vi "CoboltLaser_ResponseCheck.vi"(0 "Response":string, 1 "ExpectedResponseType":T1 items=["Any", "Digits Only", "Non-Digits Only"], 2 "ExpectedResponseMinimumLength":i32 min=0 step=1, 3 "ErrorMessage":string, 4 "GenerateErrorIfFail":bool, 5 "ErrorIn":errorcluster) -> (15 "ResponseOK":bool, 16 "Retry":bool, 19 "ErrorOut":errorcluster)   [LabVIEW 2012, in "Cobolt.lvclass"]
doc: "Use this template to build a VI to use as a subVI."
uses:
  Template/Cobolt.lvclass
  CoboltLaser_Controls/ExpectedResponseType.ctl
  Instance           1 26Saved   PR59_ResponseCheck .vi
  <vilib>/regexp/Match Regular Expression.xnode
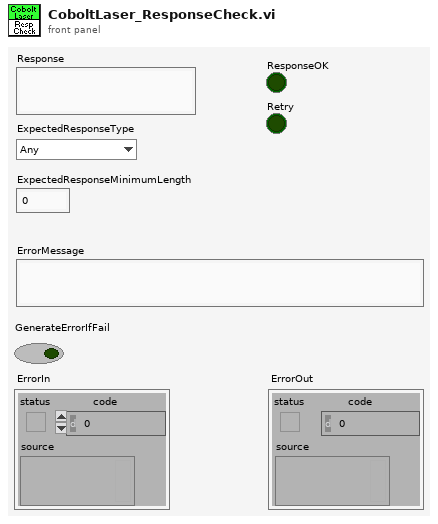
[diagram p1: front panel]
types:
  T1 = typedef "Cobolt.lvclass/ExpectedResponseType.ctl" = u16
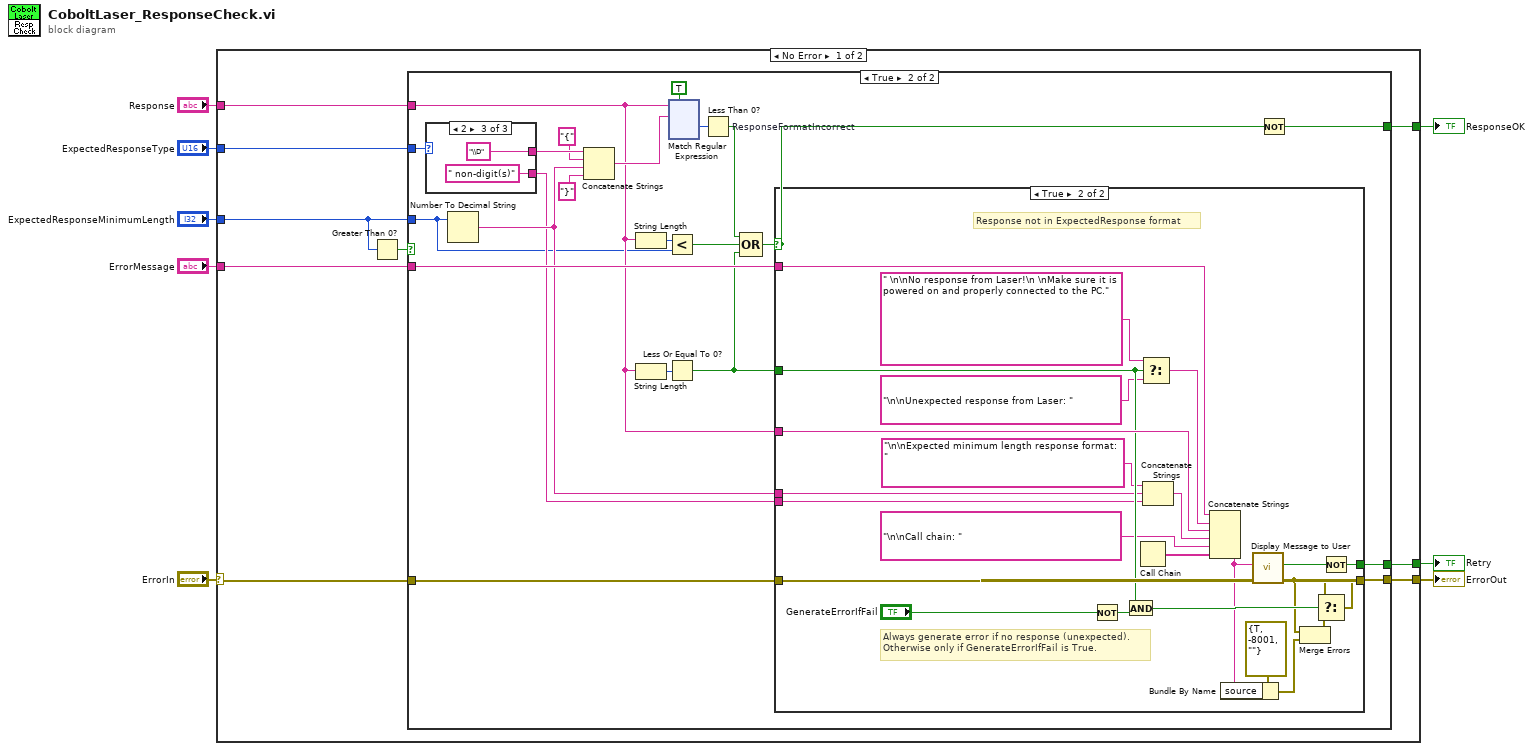
[diagram p0: block diagram]
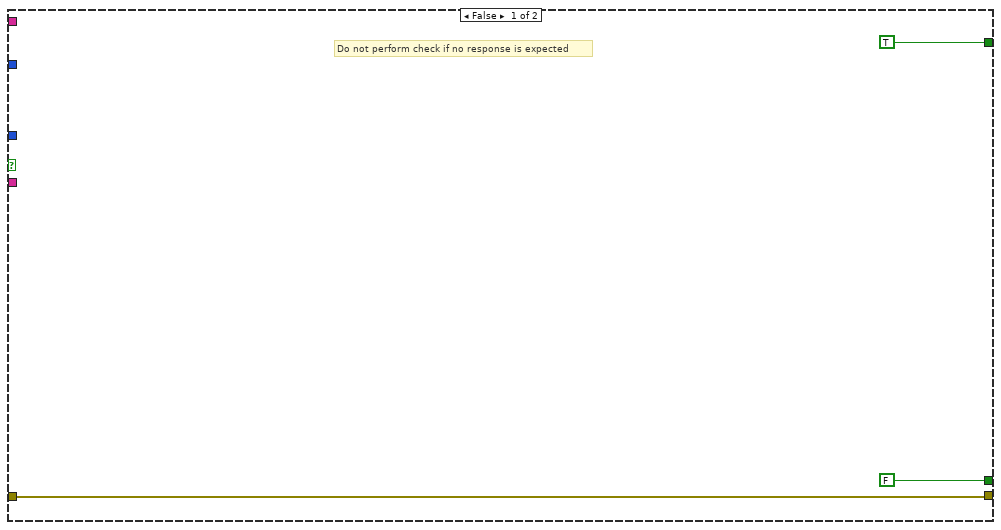
[diagram p2: hidden frame]
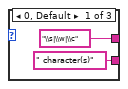
[diagram p3: hidden frame]
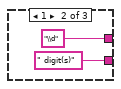
[diagram p4: hidden frame]
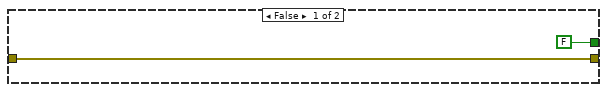
[diagram p5: hidden frame]
diagram:
  n1 = case shown="No Error" "ErrorIn" {
    selector: "ErrorIn" -> [w16 w186]
    tunnel: [w17 w186] -> w7
    tunnel: "ErrorMessage" -> [w14 _]
    tunnel: "ExpectedResponseMinimumLength" -> [w13 _]
    tunnel: "ExpectedResponseType" -> [w12 _]
    tunnel: "Response" -> [w11 _]
    tunnel: [w10 _] -> w2
    tunnel: [w9 _] -> w1
    frame No Error {
      n2 = Greater Than 0?(x=w13) -> (x > 0?=w15:bool)
      n3 = case shown="True" w15 {
        tunnel: [w18 w42] -> w17
        tunnel: w14 -> [_ w41]
        tunnel: w16 -> [w18 w40]
        tunnel: [FALSE w39] -> w9
        tunnel: w11 -> [_ w25]
        tunnel: w12 -> [_ w35]
        tunnel: w13 -> [_ w23]
        tunnel: [TRUE w29] -> w10
        frame False {
          # "Do not perform check if no response is expected"
        }
        frame True {
          n4 = case shown="2" w35 {
            tunnel: ["\\s|\\w|\\c" "\\d" "\\D"] -> w34
            tunnel: [" character(s)" " digit(s)" " non-digit(s)"] -> w27
            frame 0, Default {
            }
            frame 1 {
            }
            frame 2 {
            }
          }
          n5 = Number To Decimal String(number=w23) -> (decimal integer string=w28:string)  [unwired: 1 in]
          n6 = Concatenate Strings(w34, "{", w28, "}") -> (w31:string)
          n7 = String Length(string=w25) -> (length=w24:i32)
          n8 = String Length(string=w25) -> (length=w38:i32)
          n9 = Less?(x=w24, y=w23) -> (x < y?=w21:bool)
          n10 = Less Or Equal To 0?(x=w38) -> (x <= 0?=w22:bool)
          n11 = xnode "Match Regular Expression"("input string"=w25, "regular expression"=w31, "ignore case? (F)"=TRUE) -> ("offset past match"=w37:i32)  [unwired: 3 in, 4 out]
          n12 = Less Than 0? "ResponseFormatIncorrect"(x=w37) -> (x < 0?=w36:bool)
          n13 = Compound Arithmetic op=OR(w36, w21, w22) -> (w30:bool)
          n14 = case shown="True" w30 {
            tunnel: [w161 w183] -> w42
            tunnel: w40 -> [w161 w184]
            tunnel: w25 -> [_ w175]
            tunnel: w41 -> [_ w176]
            tunnel: [FALSE w177] -> w39
            tunnel: w22 -> [_ w174]
            tunnel: w28 -> [_ w167]
            tunnel: w27 -> [_ w165]
            frame False {
            }
            frame True {
              # "Response not in ExpectedResponse format"
              # "Always generate error if no response (unexpected).\nOtherwise only if GenerateErrorIfFail is True."
              n15 = Not(x="GenerateErrorIfFail") -> (.not. x?=w180:bool)
              n16 = And(x=w174, y=w180) -> (x .and. y?=w182:bool)
              n17 = Call Chain() -> (call chain=w171:string[])
              n18 = Select(t=" \n\nNo response from Laser!\n \nMake sure it is powered on and properly connected to the PC." ("Message"), s=w174, f="\n\nUnexpected response from Laser: " ("Message")) -> (s? t:f=w170:string)
              n19 = Concatenate Strings("\n\nExpected minimum length response format: " ("Message"), w167, w165) -> (w166:string)
              n20 = Concatenate Strings(w176, w170, w175, w166, "\n\nCall chain: " ("Message"), w171) -> (w179:string)
              n21 = Bundle By Name(cluster=errorcluster {"status"=TRUE, "code"=-8001, "source"=""} ("error out"), "source"=w179) -> (w162:errorcluster)
              n22 = call "Display Message to User"("error in (no error)"=w184, "Message"=w179) -> ("error out"=w163:errorcluster, "Continue"=w178:bool)  [unwired: 1 in, 7 out]
              n23 = Merge Errors(w163, w162) -> (w164:errorcluster)
              n24 = Select(t=w163, s=w182, f=w164) -> (s? t:f=w183:errorcluster)
              n25 = Not(x=w178) -> (.not. x?=w177:bool)
            }
          }
          n26 = Not(x=w30) -> (.not. x?=w29:bool)
        }
      }
    }
    frame Error {
    }
  }
  "ErrorOut" <- w7
  "ResponseOK" <- w2
  "Retry" <- w1
